vi "Actor Core.vi"(8 "error in":errorcluster, 11 "Device in":refnum<class "Device.lvclass">) -> (0 "error out":errorcluster, 3 "Actor out":refnum<class "Actor.lvclass">)   [LabVIEW 2014, in "DAQ Device.lvlib" / "Device.lvclass"]
doc: "(<B>Filename</B>: Actor Framework.lvlib:Actor.lvclass:Actor Core.vi)\n\nReceives messages to the actor, reacts to them, and initiates any error handling that may shut the actor down.\n\nDescendant classes may override this VI to append parallel tasks for the actor to complete while it handles messages. Overrides use the Call Parent Method node."
uses:
  Device.lvclass
  <vilib>/ActorFramework/Actor/Actor.lvclass
  <vilib>/ActorFramework/Actor/Actor.lvclass/Actor.ctl
  Device.lvclass/Device.ctl
  Devices/Configurable Device/Configurable Device.lvclass/Configurable Device.ctl
  Generic Data Update Data MSG/Generic Update Data Message.lvclass/Generic Update Data Message.ctl
  <vilib>/ActorFramework/Message Enqueuer/Message Enqueuer.lvclass/Message Enqueuer.ctl
  Generic Data Update Data MSG/Write Data.vi
  Devices/Configurable Device/Read ID.vi
  Generic Data Update Data MSG/Write ID.vi
  <vilib>/ActorFramework/Message Priority Queue/Priority Enqueue.vi
  SuperActor/Ex Nested.lvclass
  Devices/Configurable Device/Configurable Device.lvclass
  <vilib>/ActorFramework/Message Enqueuer/Message Enqueuer.lvclass
  Generic Data Update Data MSG/Generic Update Data Message.lvclass
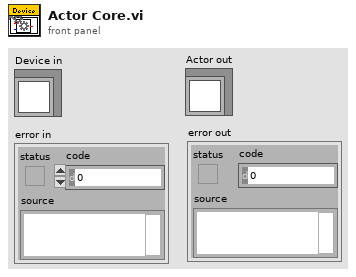
[diagram p1: front panel]
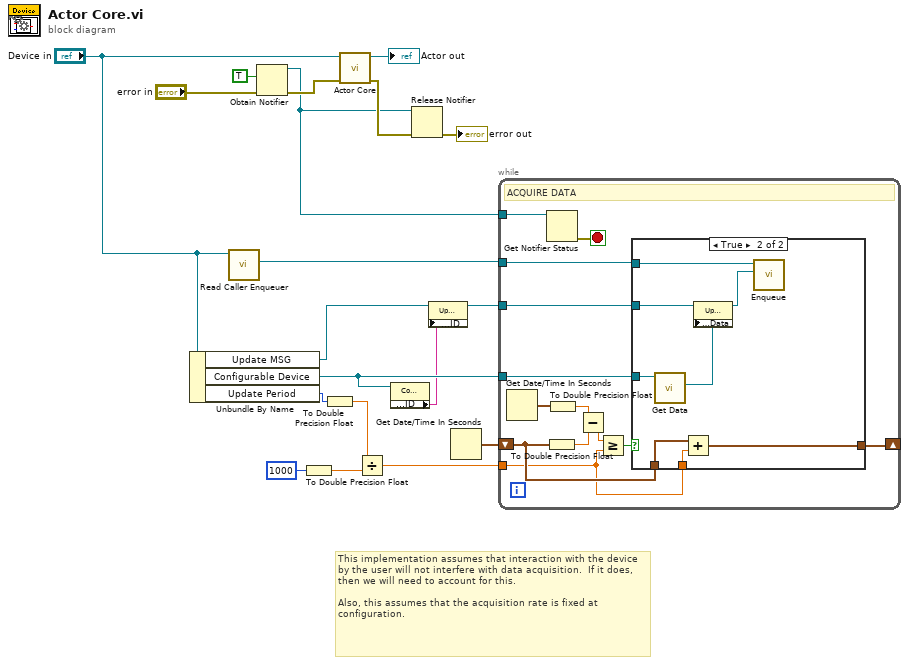
[diagram p0: block diagram]
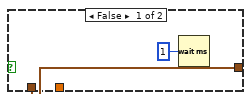
[diagram p2: hidden frame]
diagram:
  # "This implementation assumes that interaction with the device by the user will not interfere with data acquisition.  If it does, then we will need to account for this.\n\nAlso, this assumes that the acquisition rate is fixed at configuration."
  n1 = Unbundle By Name("Device in") -> ("Update MSG"=w3:refnum<class "Generic Update Data Message.lvclass">, "Configurable Device"=w8:refnum<class "Configurable Device.lvclass">, "Update Period"=w7:i32)
  n2 = call <vilib>:"Read Caller Enqueuer.vi"("Actor"="Device in") -> ("Caller Enqueuer"=w9:refnum<class "Message Enqueuer.lvclass">)  [unwired: 10 in]
  n3 = Obtain Notifier(notification data type=TRUE, error in (no error)="error in") -> (notifier out=w12:refnum<notifier>, error out=w15:errorcluster)  [unwired: 2 in, 1 out]
  n4 = To Double Precision Float(number=1000 ("y")) -> (double precision float=w5:dbl)
  n5 = To Double Precision Float(number=w7) -> (double precision float=w6:dbl)
  n6 = call-parent "Actor Core.vi"("error in"=w15, "Actor in"="Device in") -> ("error out"=w14:errorcluster, "Actor out"=→"Actor out":refnum<class "Actor.lvclass">)  [unwired: 8 in]
  n7 = Divide(x=w6, y=w5) -> (x/y=w17:dbl)
  n8 = property class="Configurable Device"(reference=w8) -> ("Accessors:ID"=w1:string)  [unwired: 1 in, 2 out]
  n9 = Release Notifier(notifier=w12, error in (no error)=w14) -> (error out=→"error out":errorcluster)  [unwired: 1 in, 2 out]
  n10 = property class="Update Data MSG"(reference=w3, "Accessors:ID"=w1) -> (reference out=w2:refnum<class "Generic Update Data Message.lvclass">)  [unwired: 1 in, 1 out]
  n11 = Get Date/Time In Seconds() -> (seconds since 1Jan1904=w18:timestamp)
  n12 = while {
    tunnel: w9 -> [w32]
    tunnel: w8 -> [w31]
    shift-right: [w23] -> _
    shift-left: w18 -> [w25]
    tunnel: w17 -> [w24]
    tunnel: w12 -> [w22]
    tunnel: w2 -> [w20]
    stop <- w21 stop-if-true
    # "ACQUIRE DATA"
    n13 = Get Date/Time In Seconds() -> (seconds since 1Jan1904=w30:timestamp)
    n14 = Get Notifier Status(notifier=w22) -> (error out=w21:errorcluster)  [unwired: 1 in, 4 out]
    n15 = To Double Precision Float(number=w25) -> (double precision float=w28:dbl)
    n16 = To Double Precision Float(number=w30) -> (double precision float=w29:dbl)
    n17 = Subtract(x=w29, y=w28) -> (x-y=w26:dbl)
    n18 = Greater Or Equal?(x=w26, y=w24) -> (x >= y?=w27:bool)
    n19 = case shown="True" w27 {
      tunnel: w32 -> [_ w42]
      tunnel: w31 -> [_ w41]
      tunnel: w25 -> [w34 w40]
      tunnel: w24 -> [_ w39]
      tunnel: [w34 w38] -> w23
      tunnel: w20 -> [_ w37]
      frame False {
        n20 = Wait (ms)(milliseconds to wait=u32 1) -> ()  [unwired: 1 out]
      }
      frame True {
        n21 = call-dynamic "Get Data.vi"("Configurable Device in"=w41) -> ("DataOut"=w36:refnum<class "Data.lvclass">)  [unwired: 8 in, 2 out]
        n22 = Add(x=w40, y=w39) -> (x+y=w38:timestamp)
        n23 = property class="Update Data MSG"(reference=w37, "Accessors:Data"=w36) -> (reference out=w35:refnum<class "Generic Update Data Message.lvclass">)  [unwired: 1 in, 1 out]
        n24 = call <vilib>:"Enqueue.vi"("Message"=w35, "Message Enqueuer in"=w42) -> ()  [unwired: 8 in, 2 out]
      }
    }
  }
